vi "Send Message.vi"(8 "error in (no error)":errorcluster, 10 "Message":string, 11 "Instrument Actor in":refnum<class "Instrument Actor.lvclass">) -> (0 "error out":errorcluster, 3 "Instrument Actor out":refnum<class "Instrument Actor.lvclass">)   [LabVIEW 2020, in "Instrument Actor.lvclass"]
uses:
  Instrument Actor.lvclass
  NHMFL_Core/Libraries/Instruments/Instrument Driver/Instrument Driver.lvclass
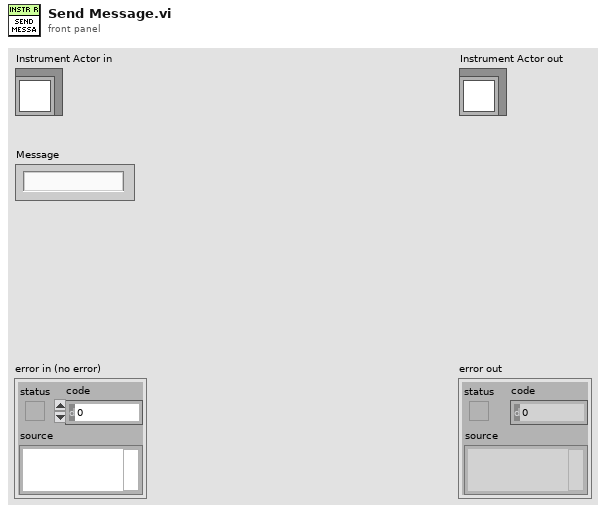
[diagram p1: front panel]
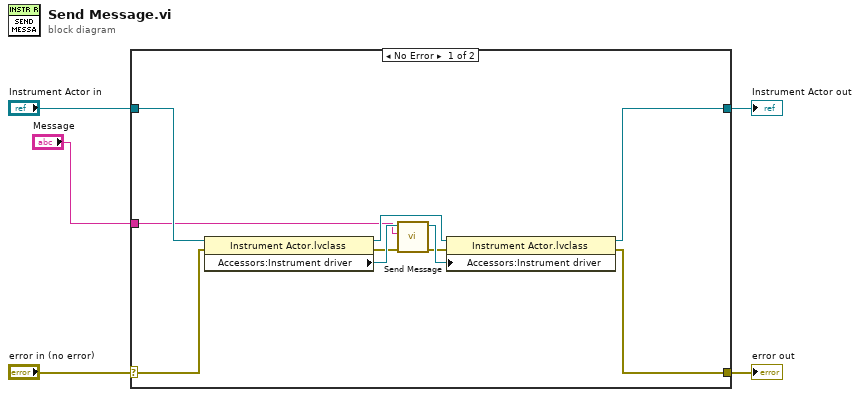
[diagram p0: block diagram]
diagram:
  n1 = case shown="No Error" "error in (no error)" {
    selector: "error in (no error)" -> [w10 w17]
    tunnel: [w9 w17] -> w4
    tunnel: [w8 w16] -> w2
    tunnel: "Instrument Actor in" -> [w7 w16]
    tunnel: "Message" -> [w6 _]
    frame No Error {
      n2 = property class="Instrument Actor.lvclass"(reference=w7, error in=w10) -> (reference out=w15:refnum<class "Instrument Actor.lvclass">, error out=w12:errorcluster, "Accessors:Instrument driver"=w14:refnum<class "Instrument Driver.lvclass">)
      n3 = call-dynamic "Send Message.vi"("error in (no error)"=w12, "Message"=w6, "Instrument Driver in"=w14) -> ("error out"=w11:errorcluster, "Instrument Driver out"=w13:refnum<class "Instrument Driver.lvclass">)  [unwired: 7 in]
      n4 = property class="Instrument Actor.lvclass"(reference=w15, error in=w11, "Accessors:Instrument driver"=w13) -> (reference out=w8:refnum<class "Instrument Actor.lvclass">, error out=w9:errorcluster)
    }
    frame Error {
    }
  }
  "error out" <- w4
  "Instrument Actor out" <- w2
